vi "I64 to JSON Value.vi"(1 "Value":i64, 2 "Name":string="hello") -> (0 "JSON Value":string)   [LabVIEW 2013, in "LV JSON.lvlib"]
uses:
  LV JSON.lvlib
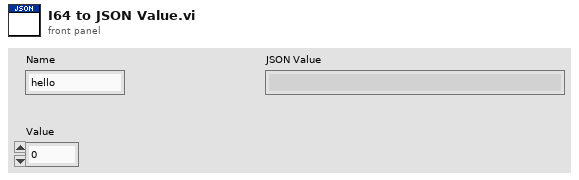
[diagram p1: front panel]
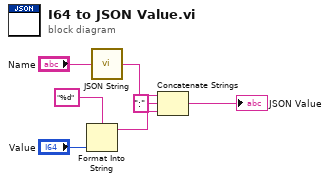
[diagram p0: block diagram]
diagram:
  n1 = Format Into String(format string="%d", "Value") -> (resulting string=w1:string)  [unwired: 2 in, 1 out]
  n2 = call "JSON String.vi"("in"="Name") -> ("out"=w6:string)
  n3 = Concatenate Strings(w6, ":" ("string"), w1) -> (→"JSON Value":string)
